vi "Enque_Message_FGV.vi"(6 "Priority":bool, 8 "error in (no error)":errorcluster, 9 "Message Data":variant, 10 "Message":string, 11 "queue Out":refnum<queue>) -> (0 "error out":errorcluster)   [LabVIEW 2024, in "Barcode_Scanner.lvlib"]
doc: "ThisVI\n------------------------------\nEnqueue Message\n------------------------------\n-Enqueue the message in message queue.\n-set Priority to true to enqueue at oposite end"
uses:
  Barcode_Scanner.lvlib
  PrivateControls/FGV_Queue_Control.ctl
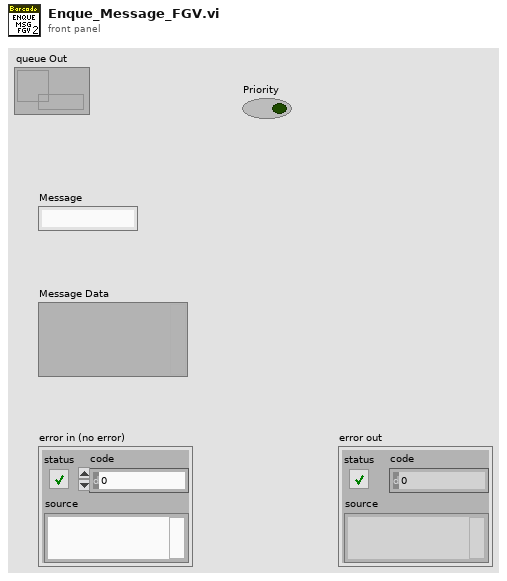
[diagram p1: front panel]
types:
  T1 = cluster{"Message":string, "Message Data":variant}
  T2 = typedef "Barcode_Scanner.lvlib/FGV_Queue_Control.ctl" = enum16{"Release", "Get", "Set"}
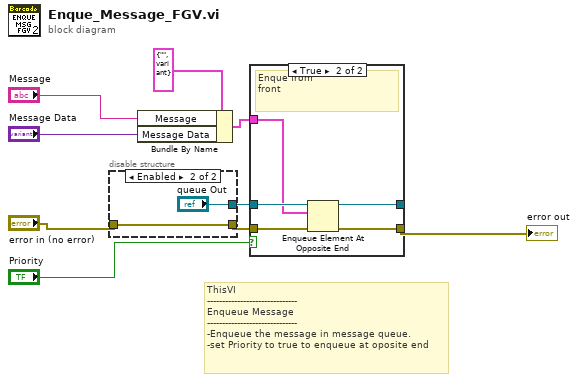
[diagram p0: block diagram]
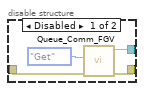
[diagram p2: hidden frame]
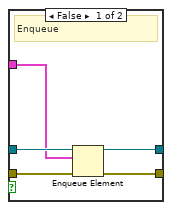
[diagram p3: hidden frame]
diagram:
  # "ThisVI\n------------------------------\nEnqueue Message\n------------------------------\n-Enqueue the message in message queue.\n-set Priority to true to enqueue at oposite end"
  n1 = disable-structure shown="Enabled" {
    disable-tunnel: [w13 "queue Out"] -> w5
    disable-tunnel: [w12 w15] -> w3
    disable-tunnel: "error in (no error)" -> [w10 w15]
    frame Disabled {
      n2 = call "Queue_Comm_FGV.vi"("error in (no error)"=w10, "Enum"=FGV_Queue_Control."Get") -> ("error Out"=w12:errorcluster, "queue Out"=w13:refnum<queue>)  [unwired: 8 in]
    }
    frame Enabled {
    }
  }
  n3 = Bundle By Name(cluster=T1 {"Message"="", "Message Data"=variant} ("element"), "Message"="Message", "Message Data"="Message Data") -> (w7:T1)
  n4 = case shown="True" "Priority" {
    tunnel: w3 -> [w20 w25]
    tunnel: [w19 w24] -> w4
    tunnel: w5 -> [w17 w23]
    tunnel: [w18 w22] -> _
    tunnel: w7 -> [w16 w21]
    frame False {
      # "Enqueue"
      n5 = Enqueue Element(queue=w17, element=w16, error in (no error)=w20) -> (queue out=w18:refnum<queue>, error out=w19:errorcluster)  [unwired: 1 in, 1 out]
    }
    frame True {
      # "Enque from\nfront"
      n6 = Enqueue Element At Opposite End(queue=w23, element=w21, error in (no error)=w25) -> (queue out=w22:refnum<queue>, error out=w24:errorcluster)  [unwired: 1 in, 1 out]
    }
  }
  "error out" <- w4
